vi "Print Console.vi"() -> ()   [LabVIEW 2010]
doc: "이 인쇄 큐 콘솔은 인쇄 작업 제출의 컨트롤을 시뮬레이션하고 처리 중인 인쇄 작업의 상태를 모니터합니다."
uses:
  Print LEDs.ctl
  Print Processing States.ctl
panel:
  out "인쇄 LED":T1={"대기 중"=TRUE, "초기화 중"=FALSE, "인쇄 중"=FALSE}
  out "큐 인쇄 작업":i32(slide) scale=0.0..25.0
  in  "큐 이벤트":bool
  in  "정지":bool
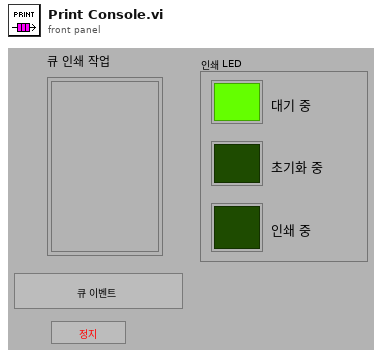
[diagram p1: front panel]
types:
  T1 = typedef "Print LEDs.ctl" = cluster{"대기 중":bool, "초기화 중":bool, "인쇄 중":bool}
  T2 = typedef "Print Processing States.ctl" = enum16{"대기", "셋업 초기화", "셋업", "인쇄 초기화", "인쇄"}
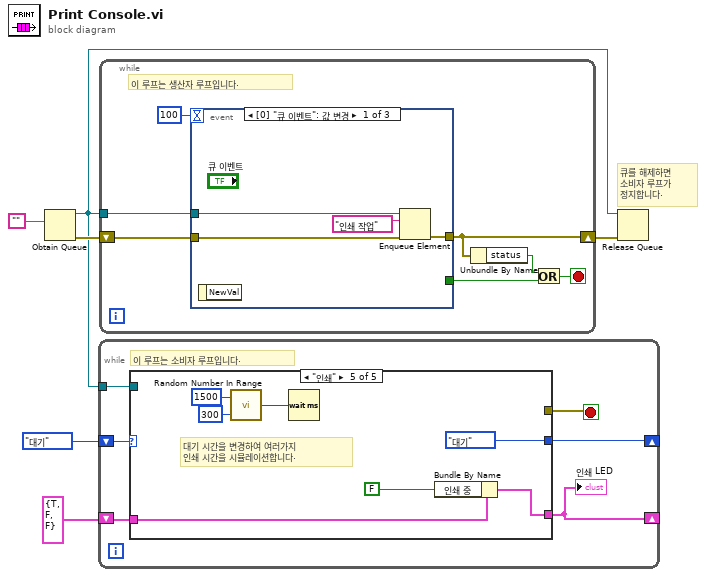
[diagram p0: block diagram]
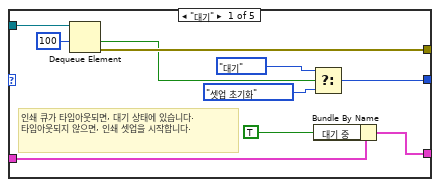
[diagram p2: hidden frame]
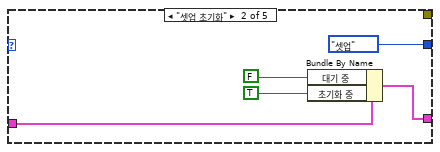
[diagram p3: hidden frame]
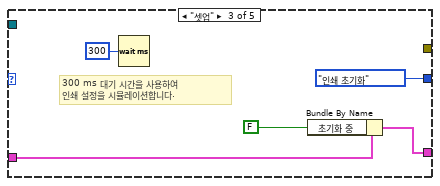
[diagram p4: hidden frame]
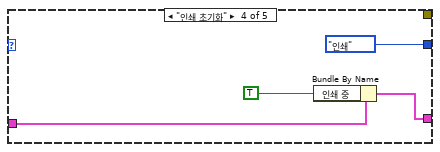
[diagram p5: hidden frame]
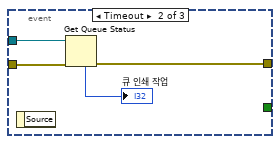
[diagram p6: hidden frame]
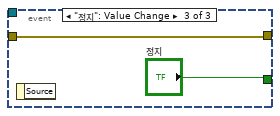
[diagram p7: hidden frame]
diagram:
  # "큐를 해제하면\n소비자 루프가\n정지합니다."
  n1 = Obtain Queue(element data type="") -> (queue out=w3:refnum<queue>, error out=w6:errorcluster)  [unwired: 4 in, 1 out]
  n2 = while {
    tunnel: w3 -> [w12]
    shift-right: [w9] -> _
    shift-left: Print_Processing_States."대기" ("Enum") -> [w11]
    shift-right: [w7] -> _
    shift-left: T1 {"대기 중"=TRUE, "초기화 중"=FALSE, "인쇄 중"=FALSE} ("Print LEDs") -> [w10]
    stop <- w8 stop-if-true
    # "이 루프는 소비자 루프입니다."
    n3 = case shown="\"인쇄\"" w11 {
      tunnel: w12 -> [w22 _ _ _ _]
      tunnel: [w21 _ _ _ _] -> w8
      tunnel: w10 -> [w16 w26 w31 w35 w42]
      tunnel: [w15 w25 w30 w34 w41] -> w7
      tunnel: [w13 Print_Processing_States."셋업" ("Enum") Print_Processing_States."인쇄 초기화" ("Enum") Print_Processing_States."인쇄" ("Enum") Print_Processing_States."대기" ("Enum")] -> w9
      frame "대기" {
        # "인쇄 큐가 타임아웃되면, 대기 상태에 있습니다. 타임아웃되지 않으면, 인쇄 셋업을 시작합니다."
        n4 = Dequeue Element(queue=w22, timeout in ms (-1)=100) -> (timed out?=w14:bool, error out=w21:errorcluster)  [unwired: 1 in, 2 out]
        n5 = Select(t=Print_Processing_States."대기" ("Enum"), s=w14, f=Print_Processing_States."셋업 초기화" ("Enum")) -> (s? t:f=w13:T2)
        n6 = Bundle By Name(cluster=w16, "대기 중"=TRUE ("Waiting for\nnew job...")) -> (w15:T1)
      }
      frame "셋업 초기화" {
        n7 = Bundle By Name(cluster=w26, "대기 중"=FALSE ("Waiting for\nnew job..."), "초기화 중"=TRUE ("Waiting for\nnew job...")) -> (w25:T1)
      }
      frame "셋업" {
        # "300 ms 대기 시간을 사용하여\n인쇄 설정을 시뮬레이션합니다."
        n8 = Wait (ms)(milliseconds to wait=u32 300) -> ()  [unwired: 1 out]
        n9 = Bundle By Name(cluster=w31, "초기화 중"=FALSE ("Waiting for\nnew job...")) -> (w30:T1)
      }
      frame "인쇄 초기화" {
        n10 = Bundle By Name(cluster=w35, "인쇄 중"=TRUE ("Waiting for\nnew job...")) -> (w34:T1)
      }
      frame "인쇄" {
        # "대기 시간을 변경하여 여러가지\n인쇄 시간을 시뮬레이션합니다."
        n11 = call "Random Number In Range.vi"("하위 리미트"=u32 300 ("Lower Limit"), "상위 리미트"=u32 1500 ("Upper Limit")) -> ("임의의 수"=w37:u32)
        n12 = Wait (ms)(milliseconds to wait=w37) -> ()  [unwired: 1 out]
        n13 = Bundle By Name(cluster=w42, "인쇄 중"=FALSE ("Waiting for\nnew job...")) -> (w41:T1)
      }
    }
    "인쇄 LED" <- w7
  }
  n14 = while {
    shift-right: [w46] -> w5
    shift-left: w6 -> [w49]
    tunnel: w3 -> [w50]
    stop <- w47 stop-if-true
    # "이 루프는 생산자 루프입니다."
    n15 = event shown="[0] \"큐 이벤트\": 값 변경" {
      selector: _ -> [_ _ _]
      dyn-events: _ -> [_ _ _]
      timeout: 100 -> [_ _ _]
      tunnel: w50 -> [w54 w56 _]
      tunnel: w49 -> [w53 w57 w59]
      tunnel: [w52 w55 w59] -> w46
      tunnel: [_ _ "정지"] -> w48
      event "큐 이벤트": Value Change {
        n16 = event-data() -> ()  [unwired: 1 in, 1 out]
        n17 = Enqueue Element(queue=w54, element="인쇄 작업", error in (no error)=w53) -> (error out=w52:errorcluster)  [unwired: 1 in, 2 out]
      }
      event Timeout {
        n18 = event-data() -> ()  [unwired: 1 in, 1 out]
        n19 = Get Queue Status(queue=w56, error in (no error)=w57) -> (error out=w55:errorcluster, # elements in queue=→"큐 인쇄 작업":i32)  [unwired: 1 in, 6 out]
      }
      event "정지": Value Change {
        n20 = event-data() -> ()  [unwired: 1 in, 1 out]
      }
    }
    n21 = Unbundle By Name(w46) -> ("status"=w45:bool)
    n22 = Or(x=w45, y=w48) -> (x .or. y?=w47:bool)
  }
  n23 = Release Queue(queue=w3, error in (no error)=w5) -> ()  [unwired: 1 in, 3 out]
